vi "First Step.vi"(8 "error in (no error)":errorcluster, 11 "Wavelength.lvclass in":refnum<class "Wavelength.lvclass">) -> (0 "error out":errorcluster, 2 "Current Position":dbl, 3 "Wavelength.lvclass out":refnum<class "Wavelength.lvclass">)   [LabVIEW 2012, in "Wavelength.lvclass"]
uses:
  Wavelength.lvclass
  Instruments/Spectrometer/Spectrometer Triax 550.lvclass
  Scanner/Scanner.lvclass
  Instruments/Spectrometer/JY-SPEX-TRIAX/JY-SPEX-TRIAX.lvlib
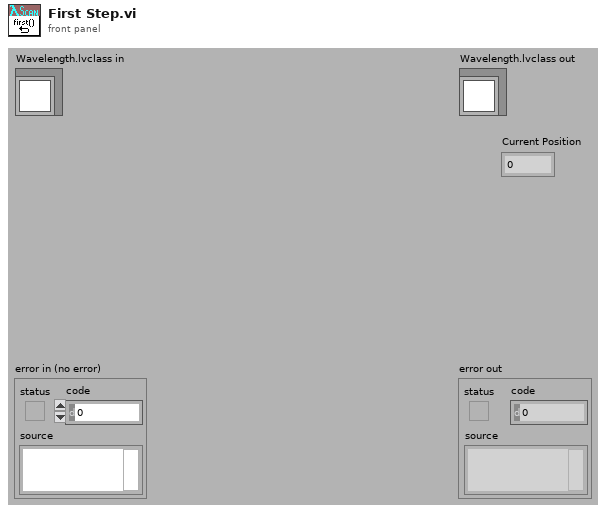
[diagram p1: front panel]
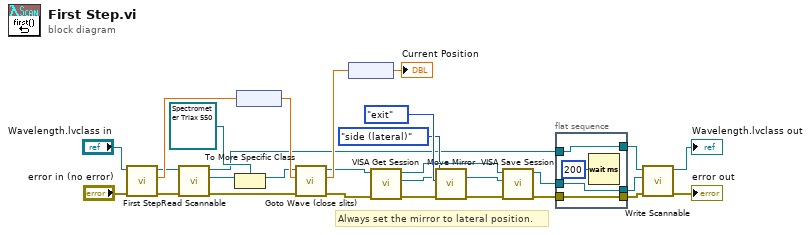
[diagram p0: block diagram]
diagram:
  # "Always set the mirror to lateral position."
  n1 = call-parent "First Step.vi"("error in (no error)"="error in (no error)", "Scanner.lvclass in"="Wavelength.lvclass in") -> ("error out"=w23:errorcluster, "Current Position"=w27:dbl, "Scanner.lvclass out"=w21:refnum<class "Wavelength.lvclass">)  [unwired: 7 out]
  n2 = call-dynamic "Read Scannable.vi"("error in (no error)"=w23, "Scanner.lvclass in"=w21) -> ("error out"=w22:errorcluster, "Scannable.lvclass"=w18:refnum<class "Scannable.lvclass">, "Scanner.lvclass out"=w6:refnum<class "Wavelength.lvclass">)  [unwired: 7 out]
  n3 = To More Specific Class(target class=refnum<class "Spectrometer Triax 550.lvclass"> refnum ("Spectrometer Triax 550.lvclass"), reference=w18) -> (specific class reference=w17:refnum<class "Spectrometer Triax 550.lvclass">)  [unwired: 1 in, 1 out]
  n4 = node(w27) -> (w24:dbl[unit])
  n5 = call "Goto Wave (close slits).vi"("error in (no error)"=w22, "Target Wavelength"=w24, "Spectrometer Triax 550 in"=w17) -> ("error out"=w9:errorcluster, "Actual Wavelength"=w25:dbl[unit], "Spectrometer Triax 550 out"=w8:refnum<class "Spectrometer Triax 550.lvclass">)  [unwired: 6 out]
  n6 = node(w25) -> (→"Current Position":dbl)
  n7 = call-dynamic "VISA Get Session.vi"("error in (no error)"=w9, "Instrument.lvclass in"=w8) -> ("error out"=w13:errorcluster, "VISA Resource Name"=w14:refnum<visa-resource-name>, "Instrument.lvclass out"=w12:refnum<class "Spectrometer Triax 550.lvclass">)  [unwired: 7 out]
  n8 = call "Move Mirror.vi"("error in (no error)"=w13, "position (side/lateral)"=enum16{"side (lateral)", "front (axial)"}."side (lateral)", "mirror (exit)"=enum16{"entrance", "exit"}."exit", "VISA resource name"=w14) -> ("error out"=w11:errorcluster, "VISA resource name out"=w10:refnum<visa-resource-name>)  [unwired: 1 in, 5 out]
  n9 = call-dynamic "VISA Save Session.vi"("error in (no error)"=w11, "VISA Resource Name"=w10, "Instrument.lvclass in"=w12) -> ("error out"=w2:errorcluster, "Instrument.lvclass out"=w4:refnum<class "Spectrometer Triax 550.lvclass">)  [unwired: 7 out]
  n10 = flat-sequence {
    tunnel: w6 -> [w32]
    tunnel: [w32] -> w5
    tunnel: w4 -> [w31]
    tunnel: [w31] -> w3
    tunnel: w2 -> [w30]
    tunnel: [w30] -> w1
    frame #0 {
      n11 = Wait (ms)(milliseconds to wait=u32 200) -> ()  [unwired: 1 out]
    }
  }
  n12 = call-dynamic "Write Scannable.vi"("error in (no error)"=w1, "Scannable.lvclass"=w3, "Scanner.lvclass in"=w5) -> ("error out"=→"error out":errorcluster, "Scanner.lvclass out"=→"Wavelength.lvclass out":refnum<class "Wavelength.lvclass">)  [unwired: 7 out]
